vi "Build.vi"(7 "channel blocks":T1[](array[typedef]) {"buffer offset" format="%d bytes"}, 8 "error in (no error)":errorcluster, 9 "dst Buffer":refnum<class "Buffer.lvclass">, 10 "src Buffer":refnum<class "DBL Pointer.lvclass">, 11 "UDP Buffer Converter in":refnum<class "UDP Buffer Converter.lvclass">) -> (0 "error out":errorcluster, 3 "UDP Buffer Converter out":refnum<class "UDP Buffer Converter.lvclass">)   [LabVIEW 2017, in "UDP.lvlib" / "UDP Buffer Converter.lvclass"]
uses:
  UDP Buffer Converter.lvclass
  Builds/Data Sharing Framework/Current/Data Sharing Framework Core/DSF Core.lvlibp/Engine/Classes/Pointer/DBL Pointer.lvclass
  Builds/Data Sharing Framework/Current/Data Sharing Framework Core/DSF Core.lvlibp/Engine/Classes/Buffer/Buffer.lvclass
  Builds/Data Sharing Framework/Current/Data Sharing Framework Core/DSF Core.lvlibp/DSF Configuration API/Public/Controls/DSF Engine Channel Configuration.ctl
  Builds/Data Sharing Framework/Current/Data Sharing Framework Core/DSF Core.lvlibp/DSF Configuration API/Public/Controls/DSF Data Type.ctl
  Builds/Data Sharing Framework/Current/Data Sharing Framework Core/DSF Core.lvlibp/Engine/Classes/Buffer Converter/Buffer Converter.lvclass
  Builds/Data Sharing Framework/Current/Data Sharing Framework Core/DSF Core.lvlibp
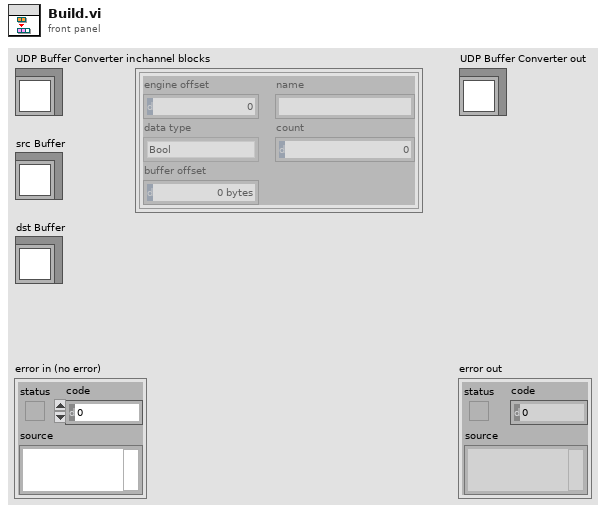
[diagram p1: front panel]
types:
  T1 = typedef "DSF Core.lvlibp/DSF Engine Channel Configuration.ctl" = cluster{"engine offset":u64, "name":string, "data type":T2, "count":u64, "buffer offset":u64}
  T2 = typedef "DSF Core.lvlibp/DSF Data Type.ctl" = enum8{"Bool", "SGL", "DBL", "I8", "I16", "I32", "I64", "U8", "U16", "U32", "U64"}
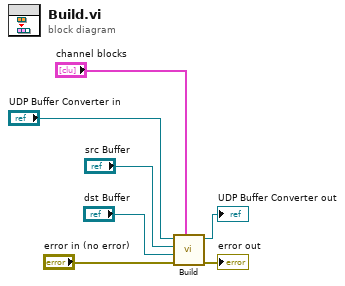
[diagram p0: block diagram]
diagram:
  n1 = call-parent "Build.vi"("channel blocks"="channel blocks", "error in (no error)"="error in (no error)", "dst Buffer"="dst Buffer", "src Buffer"="src Buffer", "Buffer Converter in"="UDP Buffer Converter in") -> ("error out"=→"error out":errorcluster, "Buffer Converter out"=→"UDP Buffer Converter out":refnum<class "UDP Buffer Converter.lvclass">)  [unwired: 5 in]
